vi "示例 2.vi"() -> ()   [LabVIEW 2021]
panel:
  out "GCD":i32
  in  "n":i32
  in  "m":i32
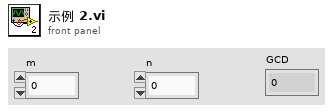
[diagram p1: front panel]
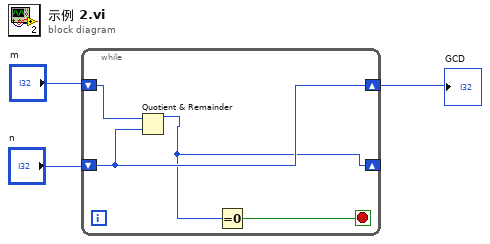
[diagram p0: block diagram]
diagram:
  n1 = while {
    shift-right: [w5] -> w1
    shift-left: "m" -> [w7]
    shift-right: [w4] -> _
    shift-left: "n" -> [w5]
    stop <- w6 stop-if-true
    n2 = Quotient & Remainder(x=w7, y=w5) -> (x-y*floor(x/y)=w4:i32)  [unwired: 1 out]
    n3 = Equal To 0?(x=w4) -> (x = 0?=w6:bool)
  }
  "GCD" <- w1
